vi "write_SCIPI+number_to_device.vi"(8 "error in (no error)":errorcluster, 9 "Numeric":dbl format="%#.6g", 10 "SCIPI":T1 items=["*IDN?", "*SAV 1", "*RCL 1", "INSTTrument CH1", "INSTTrument CH2", "INSTrument?", "MEASure:CURRent? CH1", "MEASure:CURRent? CH2", "MEASure:VOLTage? CH1", "MEASure:VOLTage? CH2", "MEASure:POWEr? CH1", "MEASure:POWEr? CH2", "CH1:CURRent?", "CH2:CURRent?", "CH1:VOLTage? ", "CH2:VOLTage? ", "OUTPut CH1,ON", "OUTPut CH1,OFF", "OUTPut CH2,ON", "OUTPut CH2,OFF", "OUTPut CH3,ON", "OUTPut CH3,OFF", "OUTPut:TRACK 0", "OUTPut:TRACK 1", "OUTPut:TRACK 2", "OUTPut:WAVE CH1,ON", "OUTPut:WAVE CH1,OFF", "OUTPut:WAVE CH2,ON", "OUTPut:WAVE CH2,OFF"], 11 "VISA":refnum<visa-resource-name>) -> (0 "error out":errorcluster, 3 "VISA resource name out":refnum<visa-resource-name>)   [LabVIEW 2020]
doc: "SCPI + numeric val"
uses:
  controls/SCPI_enum.ctl
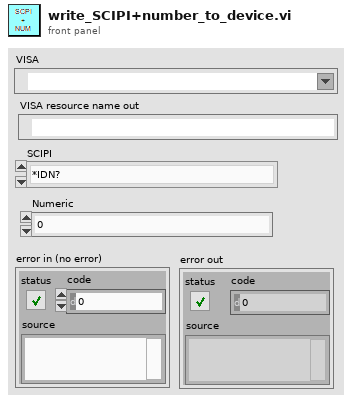
[diagram p1: front panel]
types:
  T1 = typedef "SCPI_enum.ctl" = u16
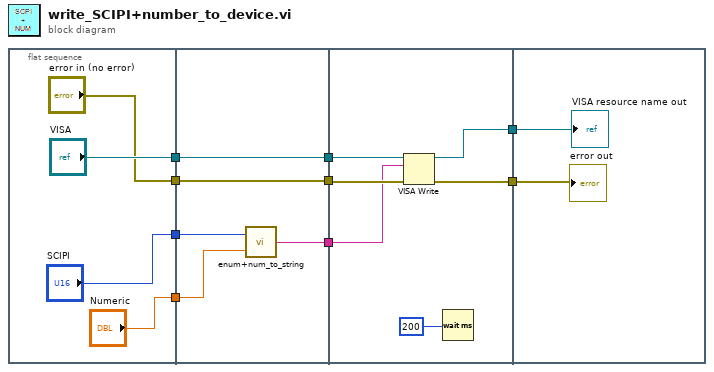
[diagram p0: block diagram]
diagram:
  n1 = flat-sequence {
    tunnel: ["VISA"] -> w7
    tunnel: ["error in (no error)"] -> w6
    tunnel: ["SCIPI"] -> w5
    tunnel: ["Numeric"] -> w4
    tunnel: w7 -> [w18]
    tunnel: [w18] -> w3
    tunnel: w6 -> [w17]
    tunnel: [w17] -> w2
    tunnel: w5 -> [w16]
    tunnel: w4 -> [w15]
    tunnel: [w14] -> w1
    tunnel: w3 -> [w23]
    tunnel: w2 -> [w22]
    tunnel: [w21] -> w9
    tunnel: [w20] -> w8
    tunnel: w1 -> [w19]
    tunnel: w9 -> [w26]
    tunnel: w8 -> [w25]
    frame #0 {
    }
    frame #1 {
      n2 = call "enum+num_to_string.vi"("Numeric"=w15, "SCIPI"=w16) -> ("concatenated string"=w14:string)
    }
    frame #2 {
      n3 = VISA Write(VISA resource name=w23, write buffer=w19, error in (no error)=w22) -> (VISA resource name out=w20:refnum<visa-resource-name>, error out=w21:errorcluster)  [unwired: 1 out]
      n4 = Wait (ms)(milliseconds to wait=u32 200) -> ()  [unwired: 1 out]
    }
    frame #3 {
      "error out" <- w26
      "VISA resource name out" <- w25
    }
  }
